vi "Config.vi"(9 "DeviceName":string="New Device", 10 "DriverID":string, 11 "DB Reference In":i32) -> ()   [LabVIEW 2020, in "ModBus TCP Master.lvlib"]
uses:
  ModBus TCP Master.lvlib
  DriverCommon/Swap.ctl
  SQLiteBase.lvlib
  DriverCommon.lvlib
panel:
  in  "Interval":u16=30
  in  "Swap":T1
  in  "Update":bool
  in  "Slave Device IP Address":string="192.168.100.254"
  in  "OK":bool
  in  "Service port":u16=502
  in  "Device ID":u16=1
  in  "Timeout":u16=1000
  # "ms"
  # "ms"
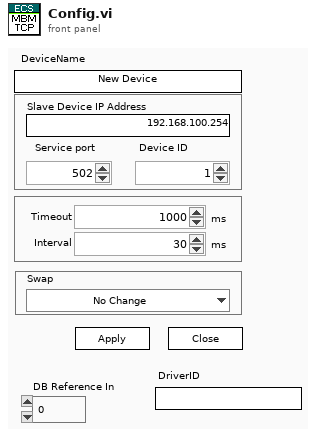
[diagram p1: front panel]
types:
  T1 = typedef "DriverCommon.lvlib/Swap.ctl" = enum16{"No Change", "Swap"}
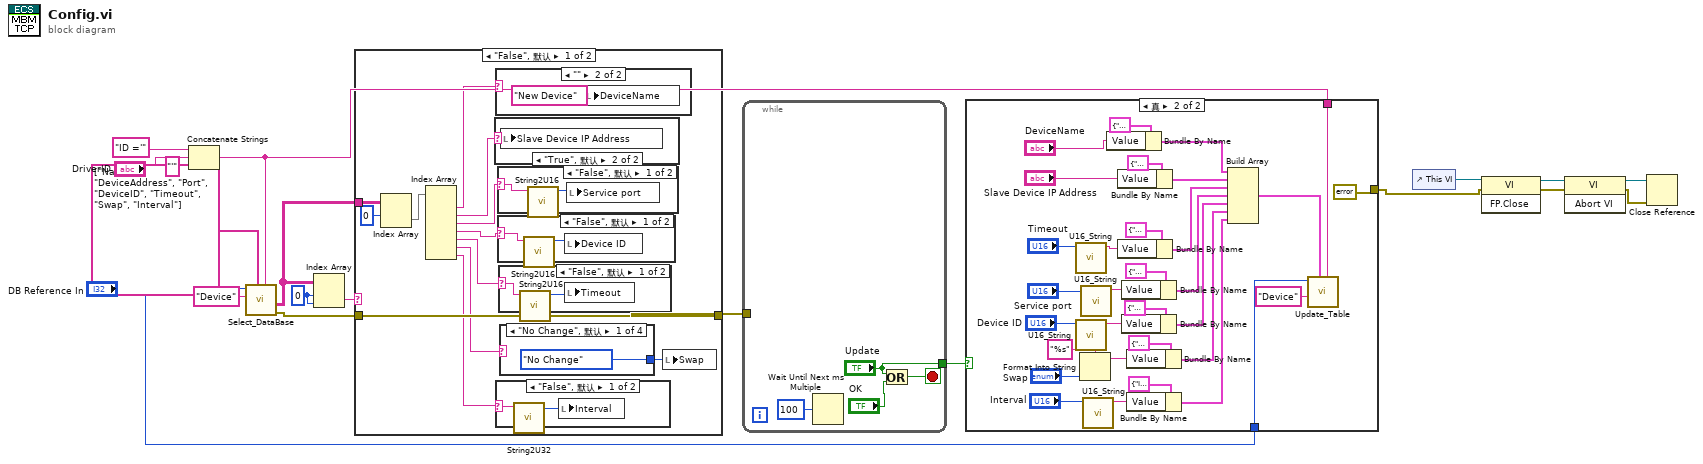
[diagram p0: block diagram]
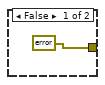
[diagram p2: hidden frame]
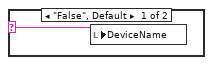
[diagram p3: hidden frame]
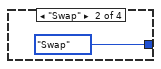
[diagram p9: hidden frame]
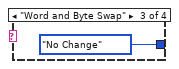
[diagram p10: hidden frame]
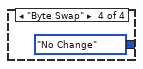
[diagram p11: hidden frame]
diagram:
  w14 = 0 ("index (row)")
  n1 = Concatenate Strings("ID ='" ("Expression"), "DriverID", "'" ("string")) -> (w8:string)
  n2 = call "Select_DataBase.vi"("Expression"=w8, "Query Columns"=string[] ["Name", "DeviceAddress", "Port", "DeviceID", "Timeout", "Swap", "Interval"], "Table name"="Device", "DB Reference In"="DB Reference In") -> ("error out"=w10:errorcluster, "Data"=w12:string[][])  [unwired: 5 in, 1 out]
  n3 = Index Array(array=w12, index (row)=w14, index (col)=w14) -> (element=w13:string)
  n4 = case shown="\"False\", 默认" w13 {
    tunnel: w12 -> [w29 _]
    tunnel: [w28 w47] -> w11
    tunnel: w10 -> [w28 w47]
    frame "False", Default {
      n5 = Index Array(array=w29, index (row)=0) -> (element=w30:string[])  [unwired: 1 in]
      n6 = Index Array(array=w30) -> (element #1=w20:string, element #2=w25:string, element #3=w24:string, element #4=w23:string, element #5=w22:string, element #6=w27:string, element #7=w21:string)  [unwired: 7 in]
      n7 = case shown="\"True\", 默认" w25 {
        selector: w25 -> [_ w42]
        frame "" {
        }
        frame "True", Default {
          n8 = local write "Slave Device IP Address"(w42) -> ()
        }
      }
      n9 = case shown="\"\"" w20 {
        selector: w20 -> [w32 _]
        frame "False", Default {
          n10 = local write "DeviceName"(w32) -> ()
        }
        frame "" {
          n11 = local write "DeviceName"("New Device" ("DeviceName")) -> ()
        }
      }
      n12 = case shown="\"False\", 默认" w21 {
        selector: w21 -> [w34 _]
        frame "False", Default {
          n13 = call "String2U32.vi"("String"=w34) -> ("U32"=w35:u32)  [unwired: 10 in]
          n14 = local write "Interval"(w35) -> ()
        }
        frame " " {
        }
      }
      n15 = case shown="\"False\", 默认" w24 {
        selector: w24 -> [w40 _]
        frame "False", Default {
          n16 = call "String2U16.vi"("String"=w40) -> ("U16"=w41:u16)  [unwired: 10 in]
          n17 = local write "Service port"(w41) -> ()
        }
        frame "" {
        }
      }
      n18 = case shown="\"False\", 默认" w23 {
        selector: w23 -> [w38 _]
        frame "False", Default {
          n19 = call "String2U16.vi"("String"=w38) -> ("U16"=w39:u16)  [unwired: 10 in]
          n20 = local write "Device ID"(w39) -> ()
        }
        frame "" {
        }
      }
      n21 = case shown="\"False\", 默认" w22 {
        selector: w22 -> [w36 _]
        frame "False", Default {
          n22 = call "String2U16.vi"("String"=w36) -> ("U16"=w37:u16)  [unwired: 10 in]
          n23 = local write "Timeout"(w37) -> ()
        }
        frame "" {
        }
      }
      n24 = case shown="\"No Change\", 默认" w27 {
        tunnel: [Swap."No Change" ("Swap") Swap."Swap" ("Swap") Swap."No Change" ("Swap") Swap."No Change" ("Swap")] -> w26
        frame "No Change", Default {
        }
        frame "Swap" {
        }
        frame "Word and Byte Swap" {
        }
        frame "Byte Swap" {
        }
      }
      n25 = local write "Swap"(w26) -> ()
    }
    frame "" {
    }
  }
  n26 = while {
    tunnel: w11 -> [_]
    tunnel: ["Update"] -> w9
    stop <- w49 stop-if-true
    n27 = Wait Until Next ms Multiple(millisecond multiple=u32 100) -> ()  [unwired: 1 out]
    n28 = Or(x="Update", y="OK") -> (x .or. y?=w49:bool)
  }
  n29 = case shown="真" w9 {
    tunnel: w8 -> [_ w74]
    tunnel: "DB Reference In" -> [_ w73]
    tunnel: [errorcluster {"status"=FALSE, "code"=0, "source"=""} ("error constant") errorcluster {"status"=FALSE, "code"=0, "source"=""} ("error constant")] -> w1
    frame False {
    }
    frame True {
      n30 = call "U16_String.vi"("U16"="Timeout") -> ("String"=w70:string)  [unwired: 10 in]
      n31 = call "U16_String.vi"("U16"="Device ID") -> ("String"=w67:string)  [unwired: 10 in]
      n32 = Format Into String(format string="%s", "Swap") -> (resulting string=w64:string)  [unwired: 2 in, 1 out]
      n33 = call "U16_String.vi"("U16"="Service port") -> ("String"=w69:string)  [unwired: 10 in]
      n34 = call "U16_String.vi"("U16"="Interval") -> ("String"=w59:string)  [unwired: 10 in]
      n35 = Bundle By Name(cluster=cluster{"column Name":string, "Value":string} {"column Name"="Name", "Value"=""} ("cell"), "Value"="DeviceName") -> (w54:cluster{"column Name":string, "Value":string})
      n36 = Bundle By Name(cluster=cluster{"column Name":string, "Value":string} {"column Name"="DeviceAddress", "Value"=""} ("cell"), "Value"="Slave Device IP Address") -> (w79:cluster{"column Name":string, "Value":string})
      n37 = Bundle By Name(cluster=cluster{"column Name":string, "Value":string} {"column Name"="Timeout", "Value"=""} ("cell"), "Value"=w70) -> (w78:cluster{"column Name":string, "Value":string})
      n38 = Bundle By Name(cluster=cluster{"column Name":string, "Value":string} {"column Name"="Port", "Value"=""} ("cell"), "Value"=w69) -> (w77:cluster{"column Name":string, "Value":string})
      n39 = Bundle By Name(cluster=cluster{"column Name":string, "Value":string} {"column Name"="DeviceID", "Value"=""} ("cell"), "Value"=w67) -> (w76:cluster{"column Name":string, "Value":string})
      n40 = Bundle By Name(cluster=cluster{"column Name":string, "Value":string} {"column Name"="Swap", "Value"=""} ("cell"), "Value"=w64) -> (w61:cluster{"column Name":string, "Value":string})
      n41 = Bundle By Name(cluster=cluster{"column Name":string, "Value":string} {"column Name"="Interval", "Value"=""} ("cell"), "Value"=w59) -> (w57:cluster{"column Name":string, "Value":string})
      n42 = Build Array(w54, w79, w78, w77, w76, w61, w57) -> (w75:cluster{"column Name":string, "Value":string}[])
      n43 = call "Update_Table.vi"("Expression"=w74, "Columns"=w75, "Table Name"="Device", "DB Reference In"=w73) -> ()  [unwired: 6 in, 2 out]
    }
  }
  n44 = control-ref of="This VI"() -> (w2:refnum<vi>)
  n45 = invoke class="VI" method="FP.Close"(reference=w2, error in=w1) -> (reference out=w3:refnum<vi>, error out=w6:errorcluster)  [unwired: 1 in, 1 out]
  n46 = invoke class="VI" method="Abort VI"(reference=w3, error in=w6) -> (reference out=w5:refnum<vi>, error out=w4:errorcluster)  [unwired: 1 in, 1 out]
  n47 = Close Reference(reference=w5, error in (no error)=w4) -> ()  [unwired: 1 out]
